vi "Selected Aircraft FGV.vi"(7 "Operation":enum16{"Get", "Set"}(ring), 8 "Error In":errorcluster, 11 "Selected Aircraft ID In":u8) -> (0 "Error Out":errorcluster, 3 "Selected Aircraft ID Out":u8)   [LabVIEW 2014]
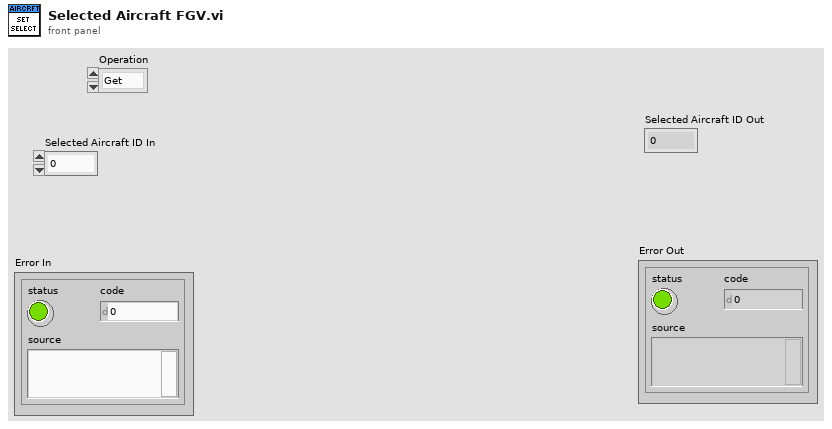
[diagram p1: front panel]
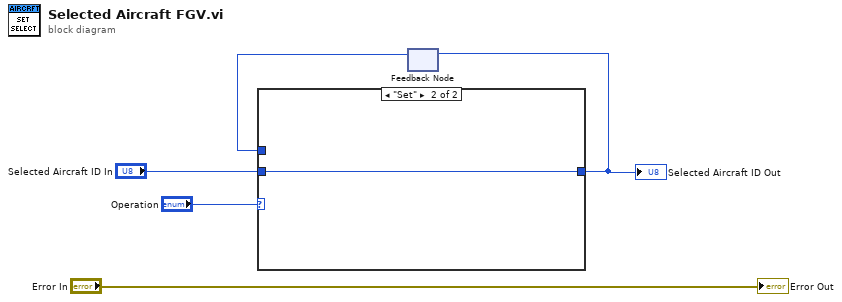
[diagram p0: block diagram]
diagram:
  n1 = feedback #1() -> (w1:u8)  [unwired: 1 in]
  n2 = case shown="\"Set\"" "Operation" {
    tunnel: "Selected Aircraft ID In" -> [_ w7]
    tunnel: [w6 w7] -> w2
    tunnel: w1 -> [w6 _]
    frame "Get", Default {
    }
    frame "Set" {
    }
  }
  "Selected Aircraft ID Out" <- w2
  n3 = feedback-in #1(w2) -> ()
  "Error Out" <- "Error In"
